vi "Generate Configuration.vi"(6 "Starting Address Offset":u16 format="%04x", 7 "Virtual Memory Unit in":refnum<class "Virtual Memory Unit.lvclass">, 8 "error in (no error)":errorcluster, 11 "1553 SubComponent in":refnum<class "1553 SubComponent.lvclass">) -> (0 "error out":errorcluster, 2 "Parameter List":string[](array[string]), 3 "1553 SubComponent out":refnum<class "1553 SubComponent.lvclass">, 4 "Next Address Offset":u16 format="%04x", 5 "Virtual Memory Unit out":refnum<class "Virtual Memory Unit.lvclass">)   [LabVIEW 2020, in "BCI-1553 API.lvlib" / "1553 SubComponent.lvclass"]
doc: "#Virtual\n\nThis does nothing. Children must override to populate the VMU with their memory config requirements. Each child should also populate and output terminal with their list of parameters that are viable targets for read/write queries."
uses:
  1553 SubComponent.lvclass
  Dependencies/Virtual Memory Unit/Virtual Memory Unit.lvclass
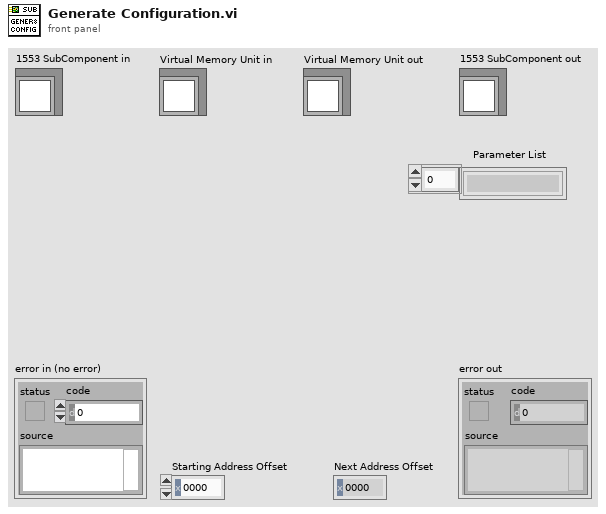
[diagram p1: front panel]
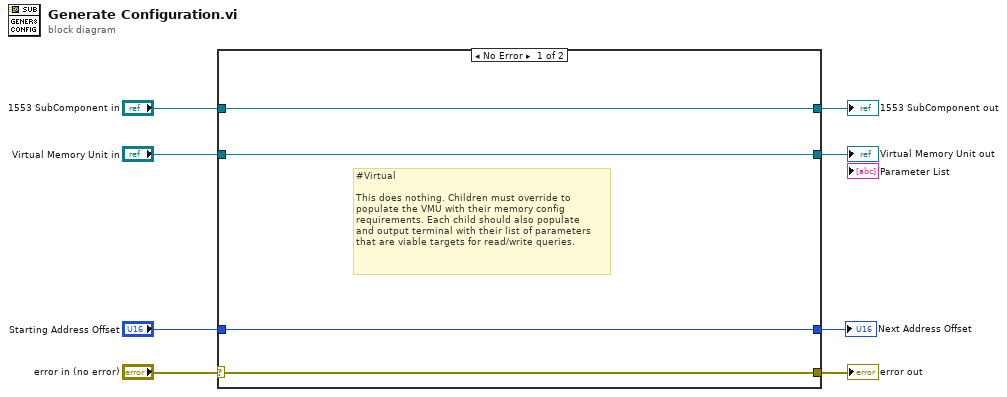
[diagram p0: block diagram]
diagram:
  n1 = case shown="No Error" "error in (no error)" {
    selector: "error in (no error)" -> [w11 w15]
    tunnel: [w11 w15] -> w7
    tunnel: [w12 w14] -> w5
    tunnel: "1553 SubComponent in" -> [w12 w14]
    tunnel: [w10 _] -> w3
    tunnel: "Virtual Memory Unit in" -> [w10 _]
    tunnel: [w9 w13] -> w2
    tunnel: "Starting Address Offset" -> [w9 w13]
    frame No Error {
      # "#Virtual\n\nThis does nothing. Children must override to\npopulate the VMU with their memory config\nrequirements. Each child should also populate\nand output terminal with their list of parameters\nthat are viable targets for read/write queries."
    }
    frame Error {
    }
  }
  "error out" <- w7
  "1553 SubComponent out" <- w5
  "Virtual Memory Unit out" <- w3
  "Next Address Offset" <- w2
